vi "Polar Plot - Auto Scale polar.vi"(10 "data":cluster{"magnitude":dbl, "phase":dbl}[](array[cluster]) {"phase" format="%0.2f"; "magnitude" format="%0.2f"}, 11 "polar attributes":T1={"maximum"=1.0, "minimum"=0.0, "clip to min"=FALSE, "log?(F)"=FALSE, "grid color"=0, "plot color"=0, "fmt and prec"={"format"=enum."Decimal", "precision"=2}, "visible section"=8} {"minimum" format="%0.2f"; "maximum" format="%0.2f"}) -> (3 "polar attributes":T1={"maximum"=1.0, "minimum"=0.0, "clip to min"=FALSE, "log?(F)"=FALSE, "grid color"=0, "plot color"=0, "fmt and prec"={"format"=enum."Decimal", "precision"=2}, "visible section"=8} {"minimum" format="%0.2f"; "maximum" format="%0.2f"})   [LabVIEW 2020]
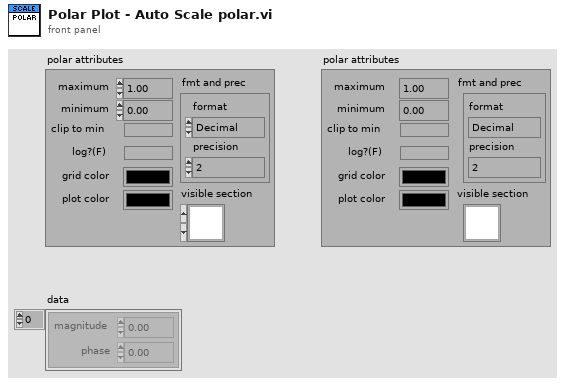
[diagram p1: front panel]
types:
  T1 = cluster{"maximum":dbl, "minimum":dbl, "clip to min":bool, "log?(F)":bool, "grid color":u32, "plot color":u32, "fmt and prec":cluster{"format":enum8{"Decimal", "Scientific", "Engineering", "Binary", "Octal", "Hex"}, "precision":u8}, "visible section":u16}
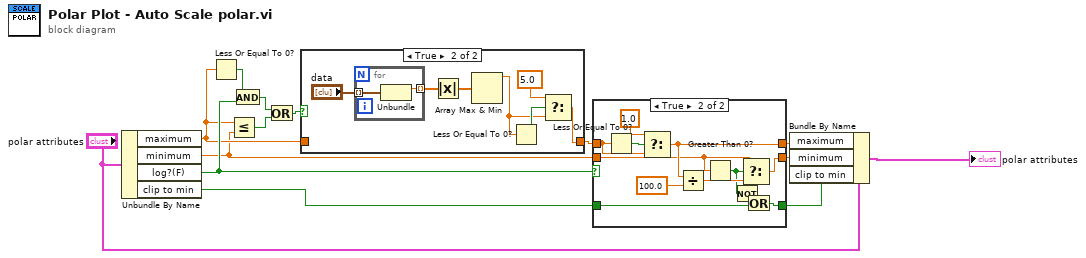
[diagram p0: block diagram]
diagram:
  n1 = Unbundle By Name("polar attributes") -> ("maximum"=w5:dbl, "minimum"=w4:dbl, "log?(F)"=w7:bool, "clip to min"=w1:bool)
  n2 = Less Or Equal To 0?(x=w5) -> (x <= 0?=w6:bool)
  n3 = Less Or Equal?(x=w5, y=w4) -> (x <= y?=w9:bool)
  n4 = And(x=w6, y=w7) -> (x .and. y?=w10:bool)
  n5 = Or(x=w10, y=w9) -> (x .or. y?=w8:bool)
  n6 = case shown="True" w8 {
    tunnel: w5 -> [w15 _]
    tunnel: [w15 w18] -> w11
    frame False {
    }
    frame True {
      n7 = for {
        tunnel: "data" -> [w24] mode=indexing
        tunnel: [w23] -> w22 mode=indexing
        n8 = Unbundle(w24) -> ("magnitude"=w23:dbl)  [unwired: 1 out]
      }
      n9 = Absolute Value(x=w22) -> (abs(x)=w17:dbl[])
      n10 = Array Max & Min(array=w17) -> (max value=w16:dbl)  [unwired: 3 out]
      n11 = Less Or Equal To 0?(x=w16) -> (x <= 0?=w20:bool)
      n12 = Select(t=5.0, s=w20, f=w16) -> (s? t:f=w18:dbl)
    }
  }
  n13 = case shown="True" w7 {
    tunnel: w4 -> [w27 w34]
    tunnel: [w27 w33] -> w12
    tunnel: w11 -> [w26 w37]
    tunnel: [w26 w35] -> w3
    tunnel: [w25 w29] -> w2
    tunnel: w1 -> [w25 w30]
    frame False {
    }
    frame True {
      n14 = Less Or Equal To 0?(x=w37) -> (x <= 0?=w38:bool)
      n15 = Select(t=1.0, s=w38, f=w37) -> (s? t:f=w35:dbl)
      n16 = Divide(x=w35, y=100.0) -> (x/y=w32:dbl)
      n17 = Greater Than 0?(x=w34) -> (x > 0?=w31:bool)
      n18 = Not(x=w31) -> (.not. x?=w28:bool)
      n19 = Select(t=w34, s=w31, f=w32) -> (s? t:f=w33:dbl)
      n20 = Or(x=w28, y=w30) -> (x .or. y?=w29:bool)
    }
  }
  n21 = Bundle By Name(cluster="polar attributes", "maximum"=w3, "minimum"=w12, "clip to min"=w2) -> (→"polar attributes":T1)
